vi "Inovance_Set_Exposure_SubVI.vi"(8 "error in (no error)":errorcluster, 9 "Exposure":dbl, 10 "OldVal":dbl, 11 "Refnum in":T1) -> (0 "error out":errorcluster, 1 "Exposure Out":dbl, 3 "Refnum out":T1)   [LabVIEW 2023, in "CameraLibrary.lvlib" / "Inovance_Camera.lvlib"]
uses:
  Inovance_Camera.lvlib
  <vilib>/userDefined/High Color/IMAQdx.ctl
  <resource>/objmgr/imaqdx.rc
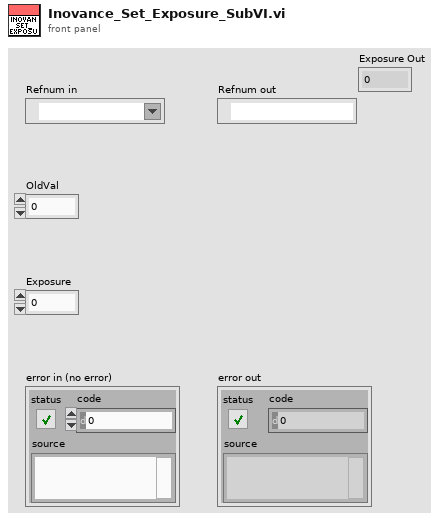
[diagram p1: front panel]
types:
  T1 = typedef "IMAQdx.ctl" = refnum<k21>
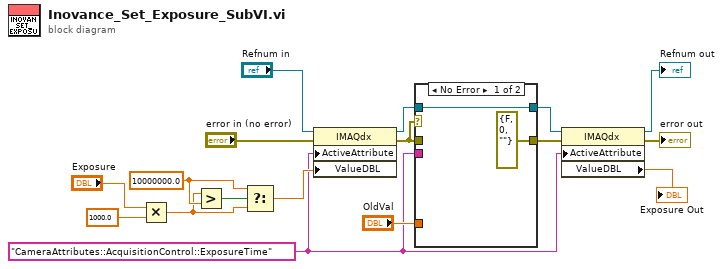
[diagram p0: block diagram]
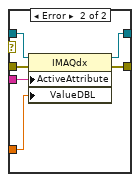
[diagram p2: hidden frame]
diagram:
  w13 = 10000000.0 ("y")
  w6 = "CameraAttributes::AcquisitionControl::ExposureTime" ("ActiveAttribute")
  n1 = Multiply(x="Exposure", y=1000.0) -> (x*y=w12:dbl)
  n2 = Greater?(x=w12, y=w13) -> (0:w11:bool)
  n3 = Select(t=w13, s=w11, f=w12) -> (s? t:f=w16:dbl)
  n4 = property class="IMAQdx"(reference="Refnum in", error in="error in (no error)", "ActiveAttribute"=w6, "ValueDBL"=w16) -> (reference out=w10:T1, error out=w17:errorcluster)
  n5 = case shown="No Error" w17 {
    tunnel: [errorcluster {"status"=FALSE, "code"=0, "source"=""} ("error constant") w23] -> w3
    tunnel: w10 -> [w18 w25]
    tunnel: "OldVal" -> [_ w20]
    tunnel: [w18 w24] -> w5
    tunnel: w17 -> [_ w22]
    tunnel: w6 -> [_ w21]
    frame No Error {
    }
    frame Error {
      n6 = property class="IMAQdx"(reference=w25, error in=w22, "ActiveAttribute"=w21, "ValueDBL"=w20) -> (reference out=w24:T1, error out=w23:errorcluster)
    }
  }
  n7 = property class="IMAQdx"(reference=w5, error in=w3, "ActiveAttribute"=w6) -> (reference out=→"Refnum out":T1, error out=→"error out":errorcluster, "ValueDBL"=→"Exposure Out":dbl)
